vi "产生电压.vi"(2 "volt":dbl, 3 "VISA error in":errorcluster, 4 "VISA resource name":refnum<visa-resource-name>) -> (0 "VISA error out":errorcluster, 1 "VISA resource name out":refnum<visa-resource-name>)   [LabVIEW 2018]
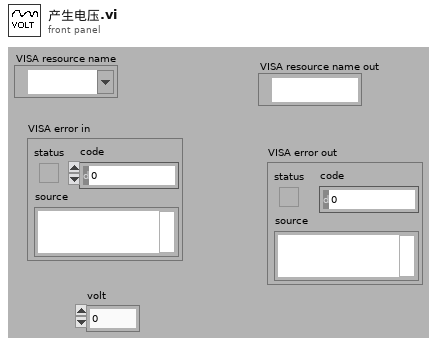
[diagram p1: front panel]
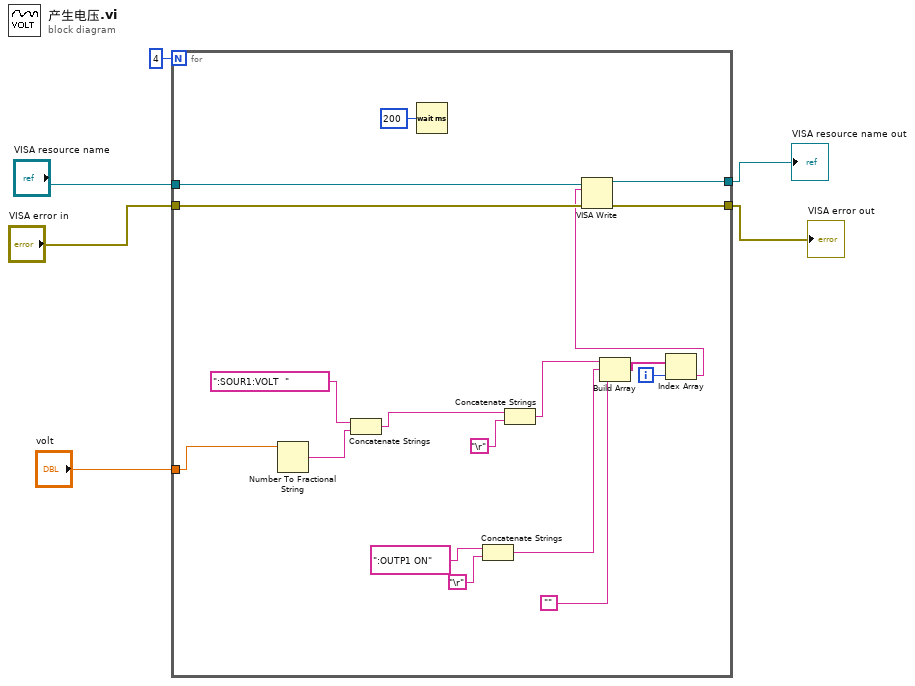
[diagram p0: block diagram]
diagram:
  n1 = for {
    N: 4 -> [_]
    tunnel: "VISA resource name" -> [w22]
    tunnel: "VISA error in" -> [w21]
    tunnel: [w20] -> w4
    tunnel: [w19] -> w3
    tunnel: "volt" -> [w10]
    i -> [w23]
    n2 = Number To Fractional String(number=w10) -> (F-format string=w12:string)  [unwired: 3 in]
    n3 = Concatenate Strings(":SOUR1:VOLT  ", w12) -> (w11:string)
    n4 = Wait (ms)(milliseconds to wait=u32 200 ("等待时间（毫秒）")) -> ()  [unwired: 1 out]
    n5 = Concatenate Strings(":OUTP1 ON", "\r") -> (w14:string)
    n6 = Concatenate Strings(w11, "\r") -> (w15:string)
    n7 = Build Array(w15, w14, "") -> (w24:string[])
    n8 = Index Array(array=w24, index=w23) -> (element=w8:string)
    n9 = VISA Write(VISA resource name=w22, write buffer=w8, error in (no error)=w21) -> (VISA resource name out=w20:refnum<visa-resource-name>, error out=w19:errorcluster)  [unwired: 1 out]
  }
  "VISA error out" <- w3
  "VISA resource name out" <- w4
